vi "x-axis.vi"(8 "error in (no error)":errorcluster, 11 "Scanner in":refnum<class "Scanner.lvclass">) -> (0 "error out":errorcluster, 1 "Label":string, 2 "Unit":string, 3 "Scanner out":refnum<class "Scanner.lvclass">)   [LabVIEW 2009, in "Scanner.lvclass"]
uses:
  Scanner.lvclass
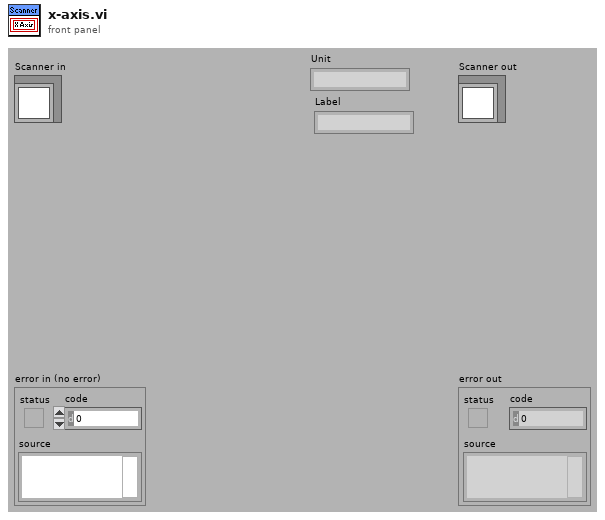
[diagram p1: front panel]
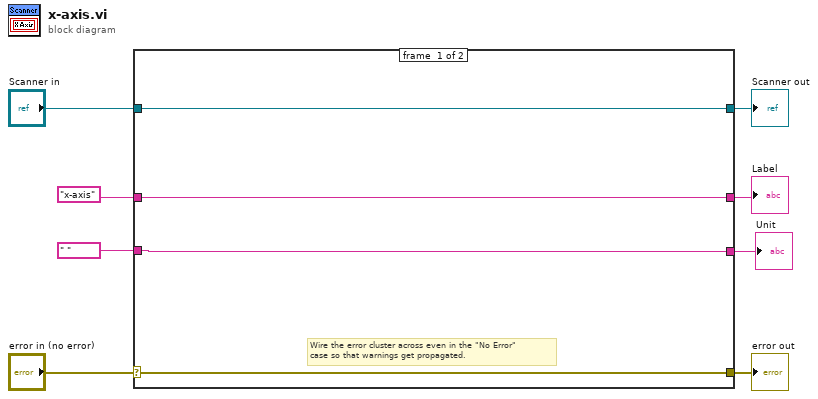
[diagram p0: block diagram]
diagram:
  n1 = case shown="Error" "error in (no error)" {
    selector: "error in (no error)" -> [w11 w16]
    tunnel: [w11 w16] -> w7
    tunnel: [w12 w15] -> w5
    tunnel: "Scanner in" -> [w12 w15]
    tunnel: [w10 w14] -> w3
    tunnel: "x-axis" ("Label") -> [w10 w14]
    tunnel: " " ("Label") -> [w9 w13]
    tunnel: [w9 w13] -> w1
    frame #0 {
      # "Wire the error cluster across even in the \"No Error\"\ncase so that warnings get propagated."
    }
    frame #1 {
    }
  }
  "error out" <- w7
  "Scanner out" <- w5
  "Label" <- w3
  "Unit" <- w1
